vi "combined_trial_wo_gas_and_laser.vi"() -> ()   [LabVIEW 2020]
uses:
  <vilib>/DAQmx/write.llb/DAQmx Write (Analog DBL 1Chan 1Samp).vi
  <vilib>/DAQmx/miscellaneous.llb/DAQmx Fill In Error Info.vi
  <instrlib>/Agilent E364X Series/Agilent E364X Series.lvlib
panel:
  out "error out":errorcluster
  out "Error Message (empty)":string
  out "error out 2":errorcluster
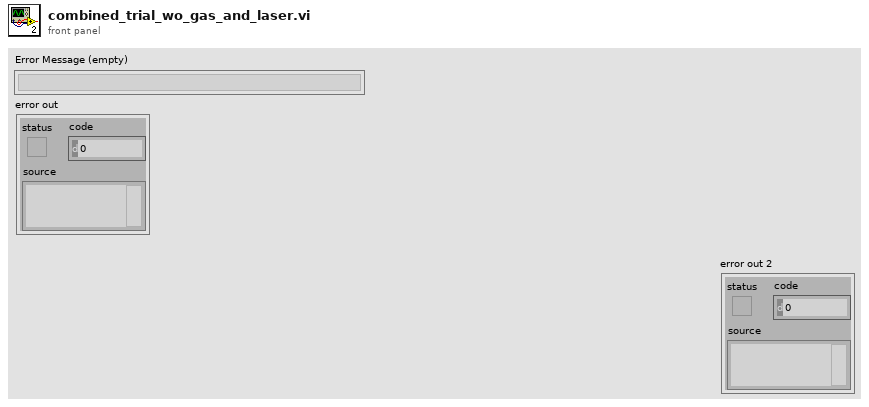
[diagram p1: front panel]
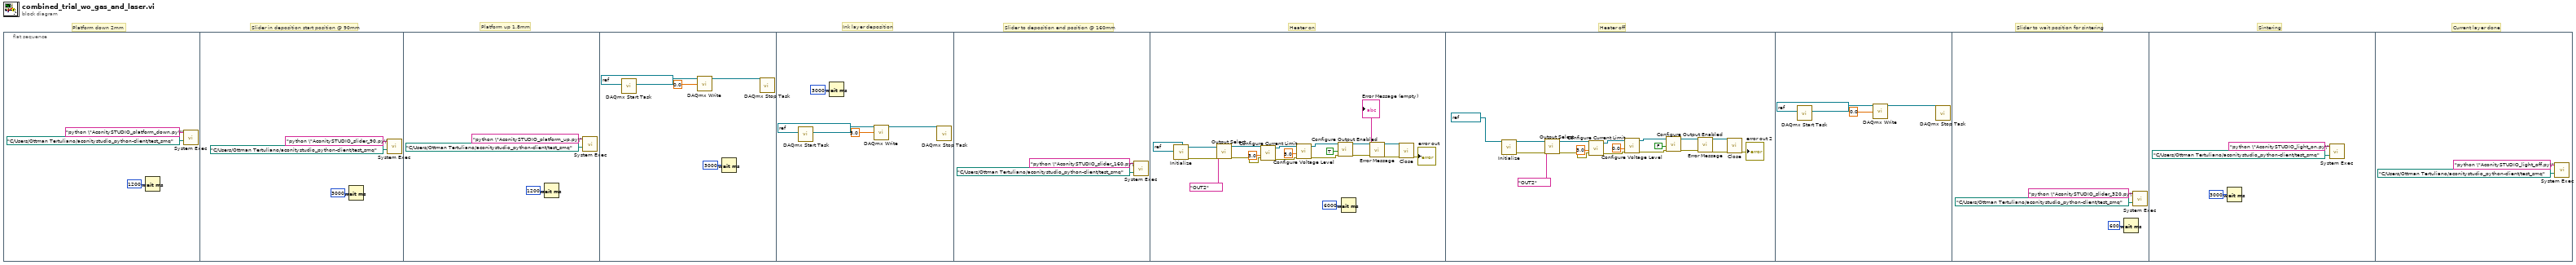
[diagram p0: block diagram]
diagram:
  # "Current layer done"
  # "Platform up 1.8mm"
  # "Sintering"
  # "Slider to wait position for sintering"
  # "Heater off"
  # "Heater on"
  # "Slider to deposition end position @ 160mm"
  # "Ink layer deposition"
  # "Slider in deposition start position @ 90mm"
  # "Platform down 2mm"
  n1 = flat-sequence {
    frame #0 {
      n2 = Wait (ms)(milliseconds to wait=u32 1200) -> ()  [unwired: 1 out]
      n3 = call <vilib>:"System Exec.vi"("working directory"=path "C:/Users/Ottman Tertuliano/aconitystudio_python-client/test_smq", "command line"="python \"AconitySTUDIO_platform_down.py\"") -> ()  [unwired: 6 in, 4 out]
    }
    frame #1 {
      n4 = Wait (ms)(milliseconds to wait=u32 3000) -> ()  [unwired: 1 out]
      n5 = call <vilib>:"System Exec.vi"("working directory"=path "C:/Users/Ottman Tertuliano/aconitystudio_python-client/test_smq", "command line"="python \"AconitySTUDIO_slider_90.py\"") -> ()  [unwired: 6 in, 4 out]
    }
    frame #2 {
      n6 = Wait (ms)(milliseconds to wait=u32 1200) -> ()  [unwired: 1 out]
      n7 = call <vilib>:"System Exec.vi"("working directory"=path "C:/Users/Ottman Tertuliano/aconitystudio_python-client/test_smq", "command line"="python \"AconitySTUDIO_platform_up.py\"") -> ()  [unwired: 6 in, 4 out]
    }
    frame #3 {
      n8 = call <vilib>:"DAQmx Start Task.vi"("task/channels in"=refnum<k21> "MyVoltageOutTask_ao0") -> ("task out"=w14:refnum<k21>)  [unwired: 13 in, 1 out]
      n9 = call-poly <vilib>:"DAQmx Write.vi"("task/channels in"=w14, "data"=0.0) -> ("task out"=w13:refnum<k21>)  [unwired: 11 in, 2 out]
      n10 = Wait (ms)(milliseconds to wait=u32 3000) -> ()  [unwired: 1 out]
      n11 = call <vilib>:"DAQmx Stop Task.vi"("task/channels in"=w13) -> ()  [unwired: 13 in, 2 out]
    }
    frame #4 {
      n12 = call <vilib>:"DAQmx Start Task.vi"("task/channels in"=refnum<k21> "MyVoltageOutTask_ao0") -> ("task out"=w19:refnum<k21>)  [unwired: 13 in, 1 out]
      n13 = Wait (ms)(milliseconds to wait=u32 3000) -> ()  [unwired: 1 out]
      n14 = call-poly <vilib>:"DAQmx Write.vi"("task/channels in"=w19, "data"=5.0) -> ("task out"=w18:refnum<k21>)  [unwired: 11 in, 2 out]
      n15 = call <vilib>:"DAQmx Stop Task.vi"("task/channels in"=w18) -> ()  [unwired: 13 in, 2 out]
    }
    frame #5 {
      n16 = call <vilib>:"System Exec.vi"("working directory"=path "C:/Users/Ottman Tertuliano/aconitystudio_python-client/test_smq", "command line"="python \"AconitySTUDIO_slider_160.py\"") -> ()  [unwired: 6 in, 4 out]
    }
    frame #6 {
      n17 = call <instrlib>:"Initialize.vi"("VISA resource name"=refnum<visa-resource-name> "COM6") -> ("error out"=w39:errorcluster, "VISA resource name out"=w40:refnum<visa-resource-name>)  [unwired: 9 in]
      n18 = call <instrlib>:"Output Select.vi"("error in (no error)"=w39, "Instrument Select (Output 1)"="OUT2", "VISA resource name"=w40) -> ("error out"=w36:errorcluster, "VISA resource name out"=w38:refnum<visa-resource-name>)  [unwired: 7 in]
      n19 = call <instrlib>:"Configure Current Limit.vi"("error in (no error)"=w36, "Current Limit (0.0 Amps)"=3.0, "VISA resource name"=w38) -> ("error out"=w34:errorcluster, "VISA resource name out"=w35:refnum<visa-resource-name>)  [unwired: 7 in]
      n20 = call <instrlib>:"Configure Voltage Level.vi"("error in (no error)"=w34, "Level (0.0 Volts)"=5.0, "VISA resource name"=w35) -> ("error out"=w32:errorcluster, "VISA resource name out"=w33:refnum<visa-resource-name>)  [unwired: 7 in]
      n21 = call <instrlib>:"Configure Output Enabled.vi"("error in (no error)"=w32, "Output Enabled (F: Off)"=TRUE, "VISA resource name"=w33) -> ("error out"=w30:errorcluster, "VISA resource name out"=w31:refnum<visa-resource-name>)  [unwired: 7 in]
      n22 = Wait (ms)(milliseconds to wait=u32 6000) -> ()  [unwired: 1 out]
      n23 = call <instrlib>:"Error Message.vi"("VISA resource name"=w31, "error in (no error)"=w30) -> ("VISA resource name out"=w28:refnum<visa-resource-name>, "Error Message (empty)"=→"Error Message (empty)":string, "error out"=w27:errorcluster)  [unwired: 9 in, 2 out]
      n24 = call <instrlib>:"Close.vi"("error in (no error)"=w27, "VISA resource name"=w28) -> ("error out"=→"error out":errorcluster)  [unwired: 9 in]
    }
    frame #7 {
      n25 = call <instrlib>:"Initialize.vi"("VISA resource name"=refnum<visa-resource-name> "COM6") -> ("error out"=w57:errorcluster, "VISA resource name out"=w58:refnum<visa-resource-name>)  [unwired: 9 in]
      n26 = call <instrlib>:"Output Select.vi"("error in (no error)"=w57, "Instrument Select (Output 1)"="OUT2", "VISA resource name"=w58) -> ("error out"=w54:errorcluster, "VISA resource name out"=w56:refnum<visa-resource-name>)  [unwired: 7 in]
      n27 = call <instrlib>:"Configure Current Limit.vi"("error in (no error)"=w54, "Current Limit (0.0 Amps)"=3.0, "VISA resource name"=w56) -> ("error out"=w52:errorcluster, "VISA resource name out"=w53:refnum<visa-resource-name>)  [unwired: 7 in]
      n28 = call <instrlib>:"Configure Voltage Level.vi"("error in (no error)"=w52, "Level (0.0 Volts)"=0.0, "VISA resource name"=w53) -> ("error out"=w50:errorcluster, "VISA resource name out"=w51:refnum<visa-resource-name>)  [unwired: 7 in]
      n29 = call <instrlib>:"Configure Output Enabled.vi"("error in (no error)"=w50, "Output Enabled (F: Off)"=FALSE, "VISA resource name"=w51) -> ("error out"=w48:errorcluster, "VISA resource name out"=w49:refnum<visa-resource-name>)  [unwired: 7 in]
      n30 = call <instrlib>:"Error Message.vi"("VISA resource name"=w49, "error in (no error)"=w48) -> ("VISA resource name out"=w47:refnum<visa-resource-name>, "error out"=w46:errorcluster)  [unwired: 9 in, 3 out]
      n31 = call <instrlib>:"Close.vi"("error in (no error)"=w46, "VISA resource name"=w47) -> ("error out"=→"error out 2":errorcluster)  [unwired: 9 in]
    }
    frame #8 {
      n32 = call <vilib>:"DAQmx Start Task.vi"("task/channels in"=refnum<k21> "MyVoltageOutTask_ao0") -> ("task out"=w63:refnum<k21>)  [unwired: 13 in, 1 out]
      n33 = call-poly <vilib>:"DAQmx Write.vi"("task/channels in"=w63, "data"=0.0) -> ("task out"=w62:refnum<k21>)  [unwired: 11 in, 2 out]
      n34 = call <vilib>:"DAQmx Stop Task.vi"("task/channels in"=w62) -> ()  [unwired: 13 in, 2 out]
    }
    frame #9 {
      n35 = Wait (ms)(milliseconds to wait=u32 600) -> ()  [unwired: 1 out]
      n36 = call <vilib>:"System Exec.vi"("working directory"=path "C:/Users/Ottman Tertuliano/aconitystudio_python-client/test_smq", "command line"="python \"AconitySTUDIO_slider_320.py\"") -> ()  [unwired: 6 in, 4 out]
    }
    frame #10 {
      n37 = Wait (ms)(milliseconds to wait=u32 3000) -> ()  [unwired: 1 out]
      n38 = call <vilib>:"System Exec.vi"("working directory"=path "C:/Users/Ottman Tertuliano/aconitystudio_python-client/test_smq", "command line"="python \"AconitySTUDIO_light_on.py\"") -> ()  [unwired: 6 in, 4 out]
    }
    frame #11 {
      n39 = call <vilib>:"System Exec.vi"("working directory"=path "C:/Users/Ottman Tertuliano/aconitystudio_python-client/test_smq", "command line"="python \"AconitySTUDIO_light_off.py\"") -> ()  [unwired: 6 in, 4 out]
    }
  }
